vi "LoadObserverControlMatrix_singleAxis_mpc.vi"(11 "NS":u16) -> (2 "SS FIFO TimeOut?":bool)   [LabVIEW 2017]
uses:
  <vilib>/rvi/interface/RandomDataEmulation/niFpgaRandomDataHandleErrors.vi
  <vilib>/rvi/DataTransferAndStorage/Container/Common/niFpgaContainerExecOnDevCompGetState.vi
  <vilib>/rvi/Emulation/niFpgaEmulationIsFPGAContextNoSignature.vi
  <vilib>/rvi/DataTransferAndStorage/Container/Common/niFpgaContainerGetUniqueNameForEmu.vi
  <vilib>/rvi/Emulation/niFpgaProcessEmulError.vi
  <vilib>/rvi/Emulation/niFpgaSctlEmulationGetInTimedLoop.vi
  <vilib>/rvi/errors/nirviReportUnexpectedCaseInternalError (U32).vi
  <vilib>/rvi/Memory/Memory_Emulation/niFpgaMemoryEmulationCacheClearOnFirstRun.vi
  <vilib>/rvi/Memory/Memory_Emulation/nirvimemoryEmulationManagerCache_MakeExclusive.vi
  <vilib>/rvi/Memory/Memory_Emulation/niFpgaMemoryEmulationValidateCache.vi
  <vilib>/rvi/Memory/Memory_Emulation/nirvimemoryEmulationManagerCache_InsertValue.vi
  <vilib>/Utility/error.llb/Clear Errors.vi
  <vilib>/rvi/Memory/Memory_Emulation/nirvimemoryEmulationManagerCache_ReleaseExclusive.vi
  <vilib>/rvi/Memory/Memory_Emulation/nirvimemoryEmulationManagerCache_GetValue.vi
  <vilib>/rvi/Memory/Memory_Emulation/nirvimemoryEmulationManagerCache_SetValue.vi
  <vilib>/rvi/Emulation/niFpgaSctlEmulationResourceMgr.vi
  <vilib>/rvi/DataTransferAndStorage/Container/XNode/niFpgaContainer.xnode
  <vilib>/rvi/interface/RandomDataEmulation/nirviRandomDataFpgaReadWriteTemplate.vi
  <vilib>/rvi/Memory/Memory_Emulation/niFpgaMemoryEmulationRefIn.vi
panel:
  # "NOTE: Ns is the number of states in the plant. The number of states in the \nobserver is Ns+1. Thus, for B, L, C, and A, we use NS+1. For K and Xss, we use Ns\nbecause the controller does not operate on the disturbance state, Xd."
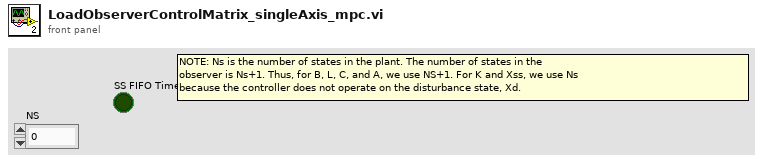
[diagram p1: front panel]
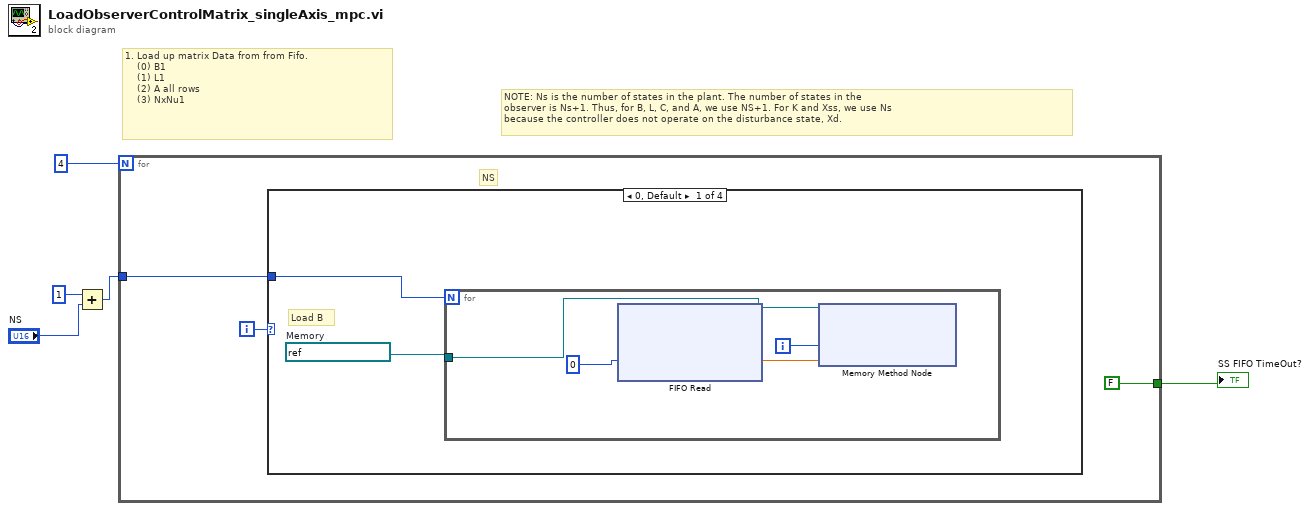
[diagram p0: block diagram]
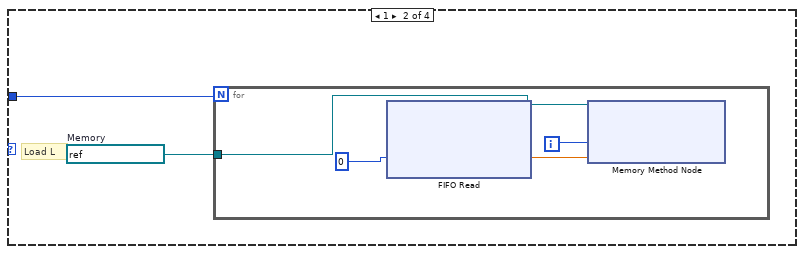
[diagram p2: hidden frame]
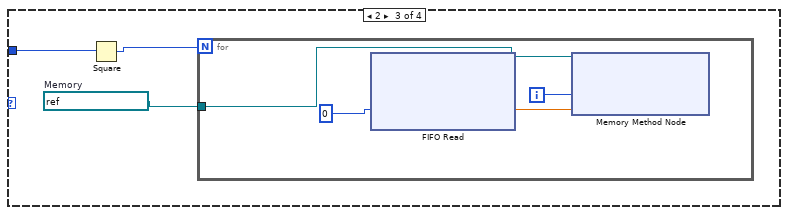
[diagram p3: hidden frame]
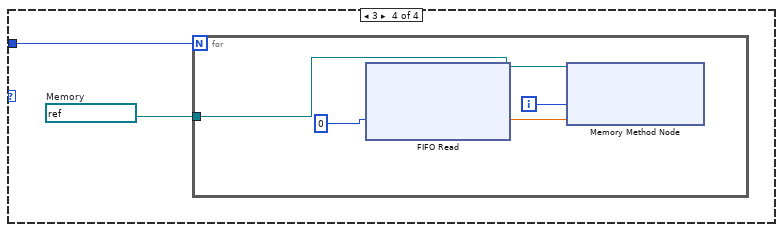
[diagram p4: hidden frame]
diagram:
  # "NOTE: Ns is the number of states in the plant. The number of states in the \nobserver is Ns+1. Thus, for B, L, C, and A, we use NS+1. For K and Xss, we use Ns\nbecause the controller does not operate on the disturbance state, Xd."
  # "1. Load up matrix Data from from Fifo.\n    (0) B1\n    (1) L1\n    (2) A all rows\n    (3) NxNu1"
  n1 = Add(x=u16 1, y="NS") -> (x+y=w1:u16)
  n2 = for {
    N: i16 4 -> [_]
    tunnel: [FALSE] -> w4
    tunnel: w1 -> [w6]
    i -> [w8]
    # "NS"
    n3 = case shown="0, Default" w8 {
      tunnel: w6 -> [w10 w16 w22 w29]
      frame 0, Default {
        w9 = refnum<k21> "Bz_FXP_col1"  # Memory
        # "Load B"
        n4 = for {
          N: w10 -> [_]
          tunnel: w9 -> [w12]
          i -> [w11]
          n5 = xnode ("FIFO Read")("Timeout"=i16 0) -> ("Element"=w14:sgl)  [unwired: 1 in, 2 out]
          n6 = xnode ("Memory Method Node")("Address"=w11, "Data"=w14, "Memory In"=w12) -> ()  [unwired: 1 out]
        }
      }
      frame 1 {
        w15 = refnum<k21> "L_FXP_col1"  # Memory
        # "Load L"
        n7 = for {
          N: w16 -> [_]
          tunnel: w15 -> [w18]
          i -> [w17]
          n8 = xnode ("FIFO Read")("Timeout"=i16 0) -> ("Element"=w20:sgl)  [unwired: 1 in, 2 out]
          n9 = xnode ("Memory Method Node")("Address"=w17, "Data"=w20, "Memory In"=w18) -> ()  [unwired: 1 out]
        }
      }
      frame 2 {
        w21 = refnum<k21> "AasCol _FXP"  # Memory
        n10 = Square(x=w22) -> (x^2=w23:u16)
        n11 = for {
          N: w23 -> [_]
          tunnel: w21 -> [w25]
          i -> [w24]
          n12 = xnode ("FIFO Read")("Timeout"=i16 0) -> ("Element"=w27:sgl)  [unwired: 1 in, 2 out]
          n13 = xnode ("Memory Method Node")("Address"=w24, "Data"=w27, "Memory In"=w25) -> ()  [unwired: 1 out]
        }
      }
      frame 3 {
        w28 = refnum<k21> "NxNu_col1"  # Memory
        n14 = for {
          N: w29 -> [_]
          tunnel: w28 -> [w31]
          i -> [w30]
          n15 = xnode ("FIFO Read")("Timeout"=i16 0) -> ("Element"=w33:sgl)  [unwired: 1 in, 2 out]
          n16 = xnode ("Memory Method Node")("Address"=w30, "Data"=w33, "Memory In"=w31) -> ()  [unwired: 1 out]
        }
      }
    }
  }
  "SS FIFO TimeOut?" <- w4
